vi "insertion_possible.vi"(8 "error in (no error)":errorcluster, 11 "DL090211FrameImageAssembler in":refnum<class "ImageAssemblerDL090211Frame.lvclass">) -> (0 "error out":errorcluster, 2 "insertion possible?":bool, 3 "DL090211FrameImageAssembler out":refnum<class "ImageAssemblerDL090211Frame.lvclass">)   [LabVIEW 2010]
uses:
  ImageAssemblerDL090211Frame.lvclass
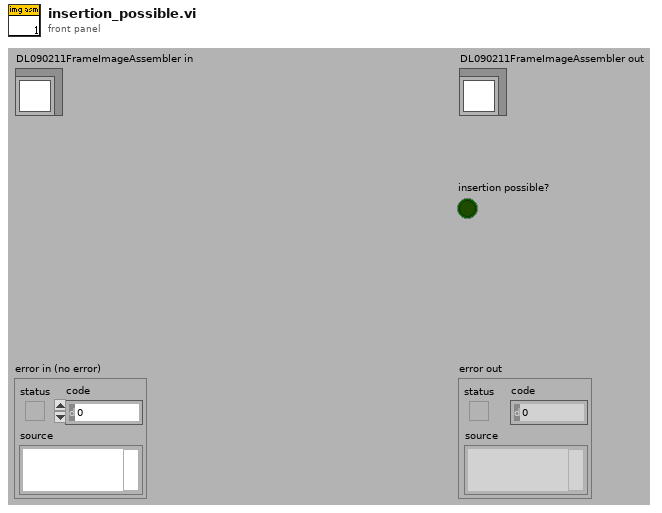
[diagram p1: front panel]
types:
  T1 = typedef "pixel_raw_data_array.ctl" = dbl[][]
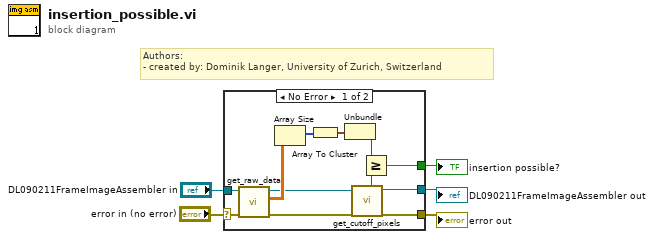
[diagram p0: block diagram]
diagram:
  # "Authors: \n- created by: Dominik Langer, University of Zurich, Switzerland"
  n1 = case shown="No Error" "error in (no error)" {
    selector: "error in (no error)" -> [w8 w19]
    tunnel: [w13 w19] -> w4
    tunnel: [w6 w18] -> w2
    tunnel: "DL090211FrameImageAssembler in" -> [w9 w18]
    tunnel: [w10 _] -> w1
    frame No Error {
      n2 = call-dynamic "get_raw_data.vi"("error in (no error)"=w8, "GenericImageAssembler.lvclass in"=w9) -> ("error out"=w14:errorcluster, "channels raw data block"=w17:T1, "GenericImageAssembler.lvclass out"=w7:refnum<class "ImageAssemblerDL090211Frame.lvclass">)  [unwired: 7 out]
      n3 = Array Size(array=w17) -> (size(s)=w16:i32[])
      n4 = Array To Cluster(array=w16) -> (cluster=w15:cluster{"[0]":i32, "[1]":i32})
      n5 = Unbundle(w15) -> ("[1]"=w11:i32)  [unwired: 1 out]
      n6 = call-dynamic "get_cutoff_pixels.vi"("error in (no error)"=w14, "DL090211FrameImageAssembler in"=w7) -> ("error out"=w13:errorcluster, "DL090211FrameImageAssembler out"=w6:refnum<class "ImageAssemblerDL090211Frame.lvclass">, "total pixels per line"=w12:i32)  [unwired: 7 out]
      n7 = Greater Or Equal?(x=w11, y=w12) -> (x >= y?=w10:bool)
    }
    frame Error {
    }
  }
  "error out" <- w4
  "DL090211FrameImageAssembler out" <- w2
  "insertion possible?" <- w1
